vi "Read Serial.vi"(8 "error in (no error)":errorcluster, 11 "VISA Reference":refnum<visa-resource-name>) -> (0 "error out":errorcluster, 2 "GetAll":T1, 3 "VISA Reference out":refnum<visa-resource-name>)   [LabVIEW 2019, in "PGC2D.lvlib"]
uses:
  PGC2D.lvlib
  sandbox/Instrument.AML.GetAll--Cluster.ctl
panel:
  out "byte count":u32=106
  out "read buffer":string
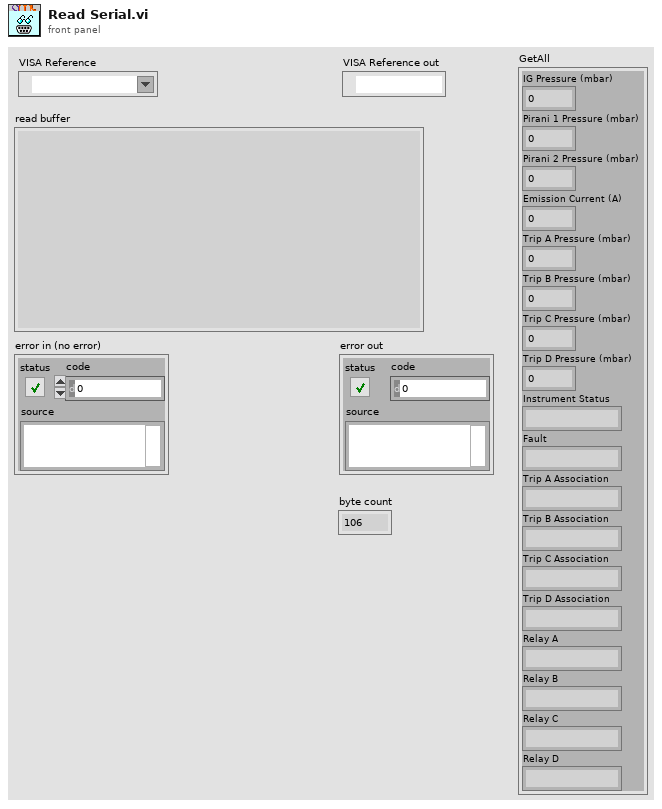
[diagram p1: front panel]
types:
  T1 = typedef "Instrument.AML.GetAll--Cluster.ctl" = cluster{"IG Pressure (mbar)":dbl, "Pirani 1 Pressure (mbar)":dbl, "Pirani 2 Pressure (mbar)":dbl, "Emission Current (A)":dbl, "Trip A Pressure (mbar)":dbl, "Trip B Pressure (mbar)":dbl, "Trip C Pressure (mbar)":dbl, "Trip D Pressure (mbar)":dbl, "Instrument Status":string, "Fault":string, "Trip A Association":string, "Trip B Association":string, "Trip C Association":string, "Trip D Association":string, "Relay A":string, "Relay B":string, "Relay C":string, "Relay D":string}
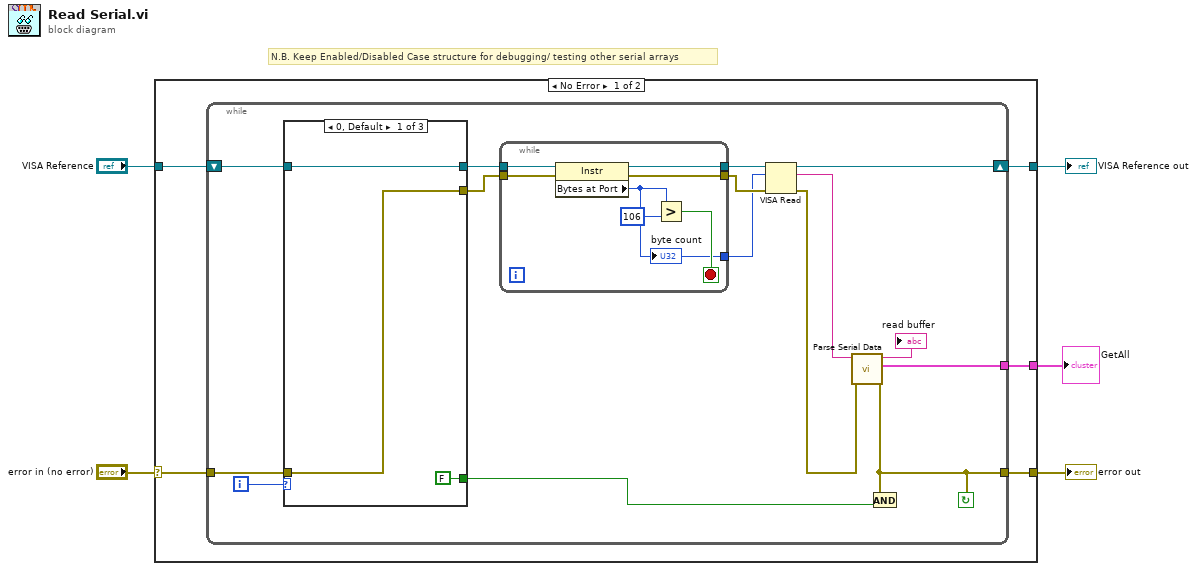
[diagram p0: block diagram]
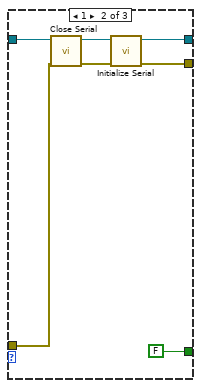
[diagram p2: hidden frame]
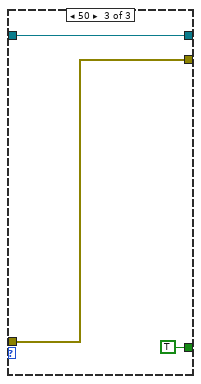
[diagram p3: hidden frame]
diagram:
  # "N.B. Keep Enabled/Disabled Case structure for debugging/ testing other serial arrays"
  n1 = case shown="No Error" "error in (no error)" {
    selector: "error in (no error)" -> [w6 w46]
    tunnel: [w7 w46] -> w5
    tunnel: [w10 w45] -> w3
    tunnel: "VISA Reference" -> [w8 w45]
    tunnel: [w9 _] -> w4
    frame No Error {
      n2 = while {
        tunnel: [w23] -> w9
        shift-right: [w25] -> w10
        shift-left: w8 -> [w15]
        tunnel: w6 -> [w17]
        tunnel: [w11] -> w7
        i -> [w19]
        stop <- w11 continue-if-true
        n3 = case shown="0, Default" w19 {
          tunnel: [w28 w34 w36] -> w18
          tunnel: w15 -> [w28 w32 w36]
          tunnel: w17 -> [w27 w31 w35]
          tunnel: [w27 w30 w35] -> w16
          tunnel: [FALSE FALSE TRUE] -> w12
          frame 0, Default {
          }
          frame 1 {
            n4 = call "Close Serial.vi"("error in (no error)"=w31, "VISA Reference"=w32) -> ("error out"=w33:errorcluster)  [unwired: 9 in]
            n5 = call "Initialize Serial.vi"("error in (no error)"=w33, "VISA resource name"=w32) -> ("error out"=w30:errorcluster, "VISA resource name out"=w34:refnum<visa-resource-name>)  [unwired: 8 in]
          }
          frame 50 {
          }
        }
        n6 = while {
          tunnel: w16 -> [w42]
          tunnel: [w41] -> w21
          tunnel: w18 -> [w44]
          tunnel: [w43] -> w22
          tunnel: [w38] -> w14
          stop <- w39 stop-if-true
          n7 = property class="Instr"(reference=w44, error in=w42) -> (reference out=w43:refnum<visa-resource-name>, error out=w41:errorcluster, "Bytes at Port"=w38:u32)
          "byte count" <- w38
          n8 = Greater?(x=w38, y=u32 106) -> (0:w39:bool)
        }
        n9 = VISA Read(VISA resource name=w22, byte count=w14, error in (no error)=w21) -> (VISA resource name out=w25:refnum<visa-resource-name>, read buffer=w20:string, error out=w13:errorcluster)  [unwired: 1 out]
        n10 = call "Parse Serial Data.vi"("error in"=w13, "Buffer in"=w20) -> ("error out"=w11:errorcluster, "cluster"=w23:T1, "Buffer out"=→"read buffer":string)  [unwired: 7 in]
        n11 = And(x=w11, y=w12) -> ()  [unwired: 1 out]
      }
    }
    frame Error {
    }
  }
  "VISA Reference out" <- w3
  "GetAll" <- w4
  "error out" <- w5
